vi "New Run From Document.vi"(7 "xwpfRun Type":refnum<class "xwpfRun.lvclass">, 8 "error in (no error)":errorcluster, 11 "Run Ref":refnum<k24>) -> (0 "error out":errorcluster, 2 "New Element Found":bool, 3 "xwpfRun out":refnum<class "xwpfRun.lvclass">)   [LabVIEW 2017, in "Word_Specific.lvlib" / "xwpfRun.lvclass"]
uses:
  xwpfRun.lvclass
  C:/Program Files (x86)/National Instruments/LabVIEW 2017/vi.lib/BenjaminR/LabVIEW NPOI/lib/NPOI 2.1.1/NPOI.OOXML.dll
  Program Files (x86)/National Instruments/LabVIEW 2017/vi.lib/BenjaminR/LabVIEW NPOI/lib/NPOI 2.1.1/NPOI.OOXML.dll
  xwpfRun.lvclass/xwpfRun.ctl
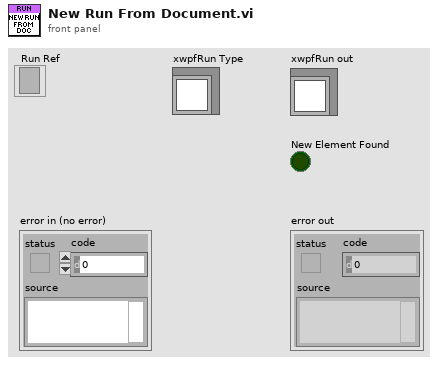
[diagram p1: front panel]
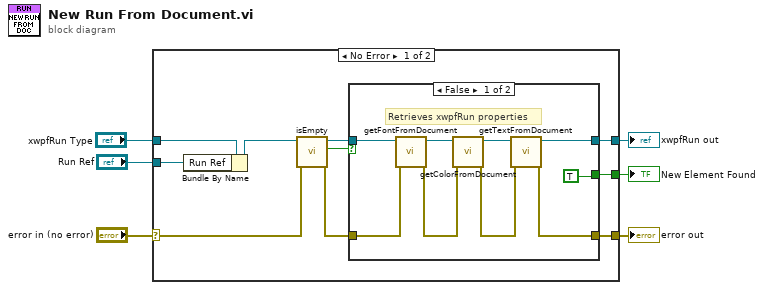
[diagram p0: block diagram]
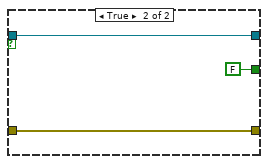
[diagram p2: hidden frame]
diagram:
  n1 = case shown="No Error" "error in (no error)" {
    selector: "error in (no error)" -> [w10 w30]
    tunnel: [w15 w30] -> w5
    tunnel: [w16 w29] -> w3
    tunnel: "xwpfRun Type" -> [w14 w29]
    tunnel: "Run Ref" -> [w12 _]
    tunnel: [w7 _] -> w1
    frame No Error {
      n2 = Bundle By Name(cluster=w14, "Run Ref"=w12) -> (w13:refnum<class "xwpfRun.lvclass">)
      n3 = call-dynamic "isEmpty.vi"("error in (no error)"=w10, "xwpfRun in"=w13) -> ("error out"=w9:errorcluster, "IsEmpty"=w8:bool, "xwpfRun out"=w11:refnum<class "xwpfRun.lvclass">)  [unwired: 7 in]
      n4 = case shown="False" w8 {
        tunnel: [w25 w28] -> w16
        tunnel: [w24 w27] -> w15
        tunnel: w11 -> [w19 w28]
        tunnel: w9 -> [w18 w27]
        tunnel: [TRUE FALSE] -> w7
        frame False {
          # "Retrieves xwpfRun properties"
          n5 = call "getFontFromDocument.vi"("error in (no error)"=w18, "xwpfRun in"=w19) -> ("error out"=w21:errorcluster, "xwpfRun out"=w23:refnum<class "xwpfRun.lvclass">)  [unwired: 8 in]
          n6 = call "getColorFromDocument.vi"("error in (no error)"=w21, "xwpfRun in"=w23) -> ("error out"=w20:errorcluster, "xwpfRun out"=w22:refnum<class "xwpfRun.lvclass">)  [unwired: 8 in]
          n7 = call "getTextFromDocument.vi"("error in (no error)"=w20, "xwpfRun in"=w22) -> ("error out"=w24:errorcluster, "xwpfRun out"=w25:refnum<class "xwpfRun.lvclass">)  [unwired: 8 in]
        }
        frame True {
        }
      }
    }
    frame Error {
    }
  }
  "error out" <- w5
  "xwpfRun out" <- w3
  "New Element Found" <- w1
